vi "Linear Programming for nD Variables.vi"() -> ()   [LabVIEW 2023]
doc: "Determines the solution of a linear programming problem of 3 or more variables and displays the solutions of the equations."
uses:
  <vilib>/Utility/error.llb/DialogType.ctl
  <vilib>/Utility/error.llb/Trim Whitespace One-Sided.vi
  <vilib>/gmath/NI_Gmath.lvlib
panel:
  in  "Subject to constraints":string[](array[string])=["-0.53*t1-1.07*t2-0.4*t3>=-180", "t1 >=30", "t2 >=30", "t3>=30", "-t1-t2-t3>=-180"]
  in  "Variables Restriction":string[](array[string])=["t1>=0", "t2>=0", "t3>= 0"]
  out "message":string
  out "C":dbl[](array[numeric])
  out "B":dbl[](array[numeric])
  out "M":dbl[][](array[numeric])
  out "Solution":dbl[](array[numeric]) format="%#.6g"
  in  "Optimization Problem":u16(ring) items=["Maximize", "Minimize"]
  in  "Objective Function":string="z=-14.14*t1+26.39*t2+13.26*t3"
  in  "Stop":bool
  out "Optimum":dbl=nan format="%#.6g"
  # "Overview: Demonstrates the use of the Linear Programming Simplex Method VI to determine the solution of a linear programming problem of 3 or more variables. \nRequirements: LabVIEW Full Development System\nInstructions: \n1. Run the VI.\n2. Change the Optimization Problem, Objective Function, and other values, and observe the Solution.\n3. Click Stop to stop the VI."
  # "Conversion"
  # "Solution"
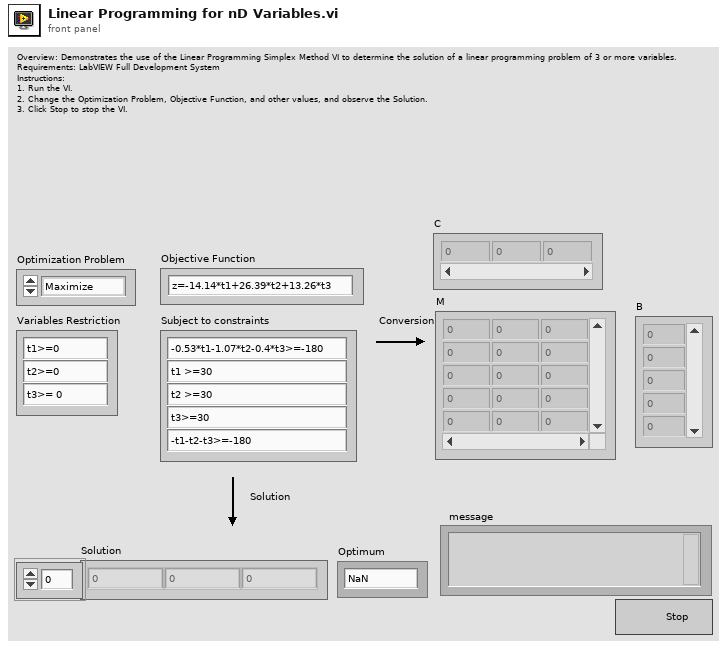
[diagram p1: front panel]
types:
  T1 = typedef "DialogType.ctl" = u16
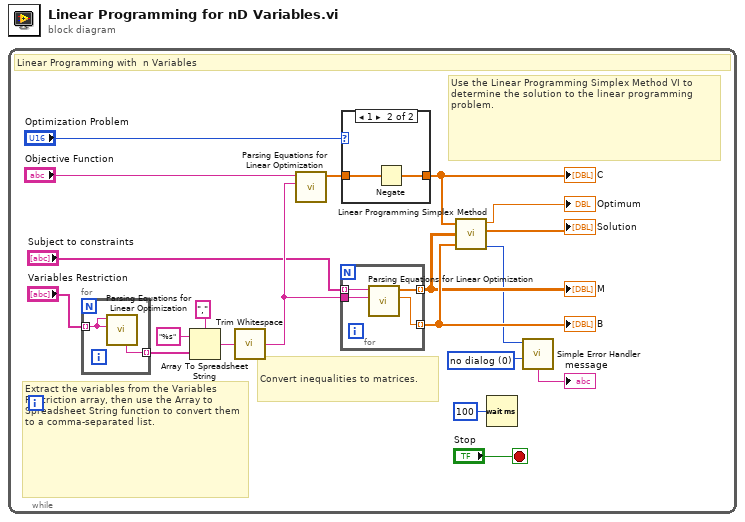
[diagram p0: block diagram]
diagram:
  n1 = while {
    stop <- "Stop" stop-if-true
    w10 = T1 0 items=["no dialog", "OK message", "continue or stop message", "OK message + warnings", "continue/stop + warnings"] ("type of dialog (OK msg:1)")
    # "Extract the variables from the Variables Restriction array, then use the Array to Spreadsheet String function to convert them to a comma-separated list."
    # "Use the Linear Programming Simplex Method VI to determine the solution to the linear programming problem."
    # "Convert inequalities to matrices."
    # "Linear Programming with  n Variables"
    n2 = for {
      tunnel: "Variables Restriction" -> [w25] mode=indexing
      tunnel: [w26] -> w6 mode=indexing
      n3 = call "Parsing Equations for Linear Optimization.vi"("Variables"=w25, "Equation"=w25) -> ("After symbol"=w26:string)  [unwired: 4 in, 5 out]
    }
    n4 = Array To Spreadsheet String(delimiter (Tab)=",", array=w6, 3:"%s" ("format string")) -> (spreadsheet string=w3:string)
    n5 = call <vilib>:"Trim Whitespace.vi"("string"=w3) -> ("trimmed string"=w2:string)  [unwired: 1 in]
    n6 = call "Parsing Equations for Linear Optimization.vi"("Variables"=w2, "Equation"="Objective Function") -> ("Vector"=w19:dbl[])  [unwired: 4 in, 5 out]
    n7 = for {
      tunnel: w2 -> [w24]
      tunnel: [w23] -> w16 mode=indexing
      tunnel: [w22] -> w17 mode=indexing
      tunnel: "Subject to constraints" -> [w21] mode=indexing
      n8 = call "Parsing Equations for Linear Optimization.vi"("Variables"=w24, "Equation"=w21) -> ("left side"=w22:dbl, "Vector"=w23:dbl[])  [unwired: 4 in, 4 out]
    }
    "B" <- w17
    "M" <- w16
    n9 = case shown="1" "Optimization Problem" {
      tunnel: w19 -> [w27 w29]
      tunnel: [w27 w28] -> w18
      frame 0, Default {
      }
      frame 1 {
        n10 = Negate(x=w29) -> (-x=w28:dbl[])
      }
    }
    "C" <- w18
    n11 = call <vilib>:"Linear Programming Simplex Method.vi"("C"=w18, "M"=w16, "B"=w17) -> ("maximum"=→"Optimum":dbl, "X"=→"Solution":dbl[], "error"=w11:i32)  [unwired: 1 out]
    n12 = Wait (ms)(milliseconds to wait=u32 100) -> ()  [unwired: 1 out]
    n13 = call <vilib>:"Simple Error Handler.vi"("error code (no error:0)"=w11, "type of dialog (OK msg:1)"=w10) -> ("message"=→"message":string)  [unwired: 3 in, 4 out]
  }
